vi "Agilent SNA Read Sweep Time.vi"(4 "Passthrough (T)":bool=TRUE, 6 "Channel":i8=1 min=1 max=99 step=1, 7 "Agilent SNA & SWP":T1, 8 "error in (no error)":errorcluster, 11 "VISA Resource Names":T2) -> (0 "error out":errorcluster, 2 "Sweep Time, s":dbl=3000.0, 3 "dup VISA Resource Name":T2)   [LabVIEW 2011]
doc: "This Vi for the HP8753B Network Analyzer is used to set averaging, smoothing, and the IF bandwidth."
uses:
  TypeDefs/Agilent SNA VISA.ctl
  TypeDefs/Agilent SNA Instrument Info.ctl
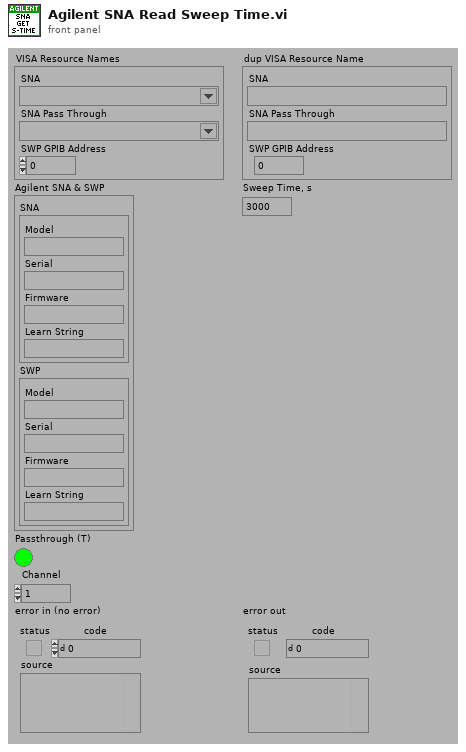
[diagram p1: front panel]
types:
  T1 = typedef "Agilent SNA Instrument Info.ctl" = cluster{"SNA":cluster{"Model":string, "Serial":string, "Firmware":string, "Learn String":string}, "SWP":cluster{"Model":string, "Serial":string, "Firmware":string, "Learn String":string}}
  T2 = typedef "Agilent SNA VISA.ctl" = cluster{"SNA":refnum<visa-resource-name>, "SNA Pass Through":refnum<visa-resource-name>, "SWP GPIB Address":i32}
  T3 = typedef "Agilent SNA Model.ctl" = enum16{"Not Supported", "8757X"}
  T4 = typedef "Agilent SNA SWP Model.ctl" = enum16{"Not Supported", "836XXX", "8375XX", "E82X7D"}
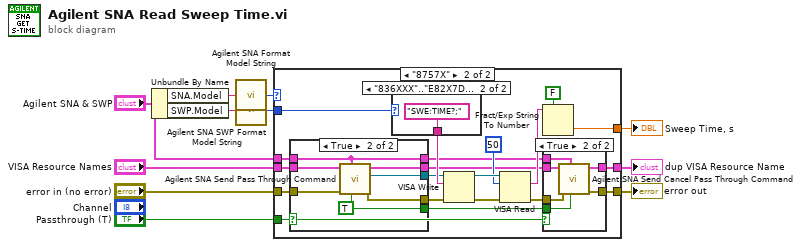
[diagram p0: block diagram]
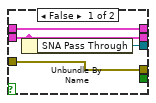
[diagram p3: hidden frame]
diagram:
  n1 = Unbundle By Name("Agilent SNA & SWP") -> ("SNA.Model"=w8:string, "SWP.Model"=w5:string)
  n2 = call "Agilent SNA Format Model String.vi"("Model String"=w8) -> ("Model"=w7:T3)
  n3 = call "Agilent SNA SWP Format Model String.vi"("Model String"=w5) -> ("Model"=w4:T4)
  n4 = case shown="\"8757X\"" w7 {
    tunnel: "error in (no error)" -> [w13 w16]
    tunnel: [w13 w25] -> w10
    tunnel: [_ w29] -> w9
    tunnel: "Agilent SNA & SWP" -> [_ w19]
    tunnel: w4 -> [_ w27]
    tunnel: [w12 w24] -> w3
    tunnel: "VISA Resource Names" -> [w12 w18]
    tunnel: "Passthrough (T)" -> [_ w14]
    frame "Not Supported" {
    }
    frame "8757X" {
      n5 = case shown="True" w14 {
        tunnel: [w35 w44] -> w20
        tunnel: w16 -> [w36 w43]
        tunnel: w18 -> [w34 w42]
        tunnel: [w36 w41] -> w21
        tunnel: w19 -> [w37 w38]
        tunnel: [w34 w40] -> w22
        tunnel: [_ w39] -> w15
        tunnel: [w37 w38] -> w17
        frame False {
          n6 = Unbundle By Name(w34) -> ("SNA Pass Through"=w35:refnum<visa-resource-name>)
        }
        frame True {
          w39 = TRUE ("SCPI? (F)")
          n7 = call "Agilent SNA Send Pass Through Command.vi"("SCPI? (F)"=w39, "Agilent SNA & SWP"=w38, "error in (no error)"=w43, "VISA Resource Names"=w42) -> ("error out"=w41:errorcluster, "SNA Pass Through"=w44:refnum<visa-resource-name>, "dup VISA Resource Names"=w40:T2)  [unwired: 5 out]
        }
      }
      n8 = case shown="\"836XXX\"..\"E82X7D\"" w27 {
        tunnel: [_ "SWE:TIME?;"] -> w26
        frame "Not Supported" {
        }
        frame "836XXX".."E82X7D" {
        }
      }
      n9 = VISA Write(VISA resource name=w20, write buffer=w26, error in (no error)=w21) -> (VISA resource name out=w33:refnum<visa-resource-name>, error out=w31:errorcluster)  [unwired: 1 out]
      n10 = VISA Read(VISA resource name=w33, byte count=u32 50, error in (no error)=w31) -> (read buffer=w28:string, error out=w23:errorcluster)  [unwired: 2 out]
      n11 = Fract/Exp String To Number(use system decimal point (T)=FALSE, string=w28) -> (number=w29:dbl)  [unwired: 3 out]
      n12 = case shown="True" w14 {
        tunnel: [w46 w52] -> w25
        tunnel: w22 -> [w45 w51]
        tunnel: w23 -> [w46 w50]
        tunnel: w15 -> [_ w49]
        tunnel: [w45 w48] -> w24
        tunnel: w17 -> [_ w47]
        frame False {
        }
        frame True {
          n13 = call "Agilent SNA Send Cancel Pass Through Command.vi"("SCPI? (F)"=w49, "Agilent SNA & SWP"=w47, "error in (no error)"=w50, "VISA Resource Names"=w51) -> ("error out"=w52:errorcluster, "dup VISA Resource Names"=w48:T2)  [unwired: 6 out]
        }
      }
    }
  }
  "error out" <- w10
  "dup VISA Resource Name" <- w3
  "Sweep Time, s" <- w9
